vi "can_test.vi"() -> ()   [LabVIEW 2020]
uses:
  <vilib>/xnet/xnet.llb/XNET Frame CAN.ctl
  <vilib>/xnet/xnet.llb/XNET Frame Type CAN.ctl
  <vilib>/xnet/xnet.llb/XNET Create Session (Frame Output Stream).vi
  <vilib>/xnet/xnet.llb/XNET Write (Frame CAN).vi
  <resource>/objmgr/xnet.rc
panel:
  out "Array 2":T1[](array[typedef]) {"payload" format="%x"; "timestamp" format="%<%.7X\n%x>T"; "type" items=["CAN Data"=0, "CAN Remote"=1, "CAN Bus Error"=2, "CAN 2.0 Data"=8, "CAN FD Data"=16, "CAN FD+BRS Data"=24, "J1939 Data"=192, "Delay"=224, "Log Trigger"=225, "Start Trigger"=226]; "identifier" format="%x"}
  out "Array":T1[](array[typedef]) {"payload" format="%x"; "timestamp" format="%<%.7X\n%x>T"; "type" items=["CAN Data"=0, "CAN Remote"=1, "CAN Bus Error"=2, "CAN 2.0 Data"=8, "CAN FD Data"=16, "CAN FD+BRS Data"=24, "J1939 Data"=192, "Delay"=224, "Log Trigger"=225, "Start Trigger"=226]; "identifier" format="%x"}
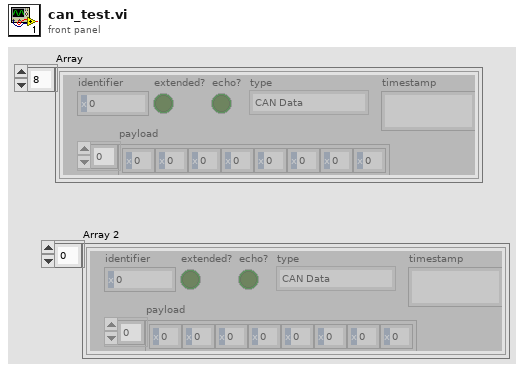
[diagram p1: front panel]
types:
  T1 = typedef "XNET Frame CAN.ctl" = cluster{"timestamp":timestamp, "payload":u8[], "identifier":u32, "type":T2, "extended?":bool, "echo?":bool}
  T2 = typedef "XNET Frame Type CAN.ctl" = u8
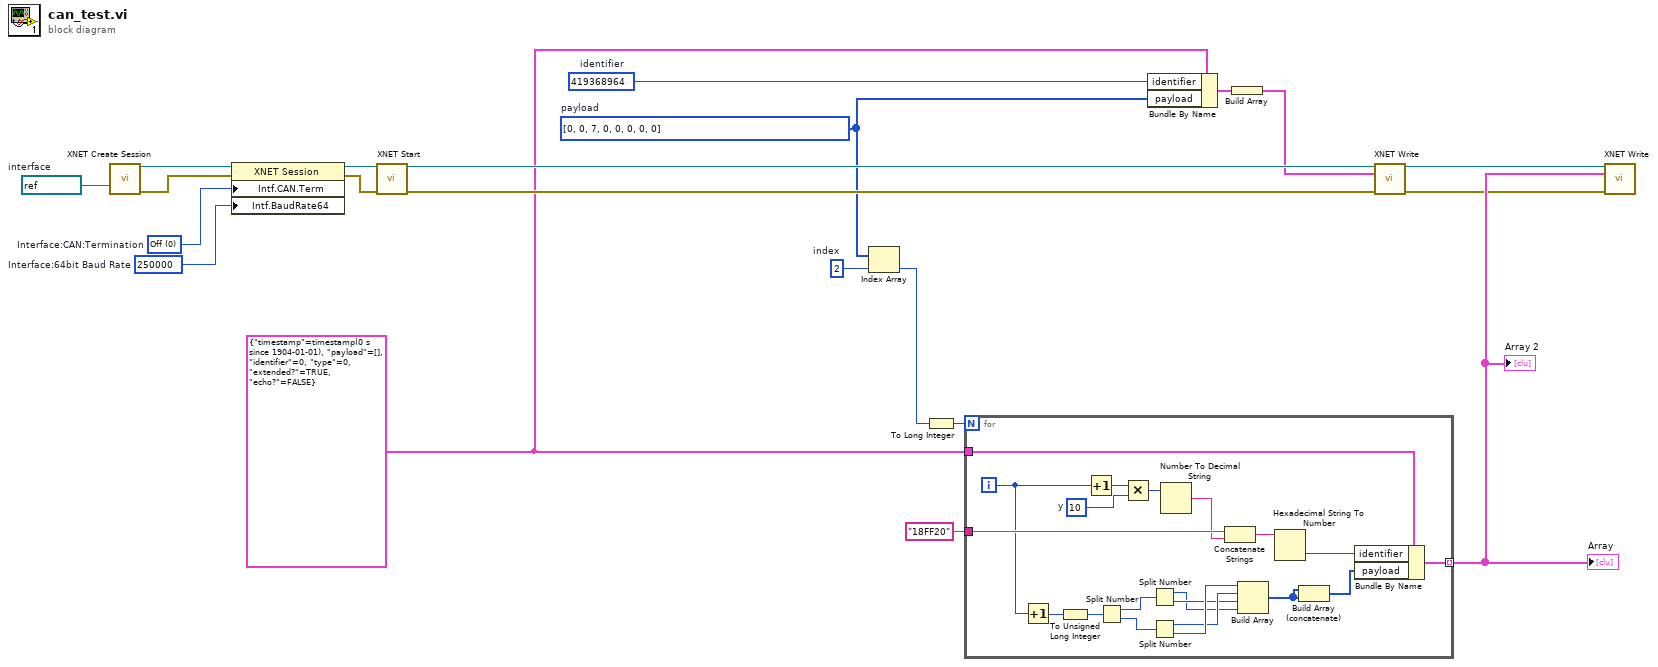
[diagram p0: block diagram]
diagram:
  w3 = 2  # index
  w4 = u8[] [0, 0, 7, 0, 0, 0, 0, 0]  # payload
  w7 = u32 419368964  # identifier
  w17 = u32 0 items=["Off", "On"]  # Interface:CAN:Termination
  w18 = u64 250000  # Interface:64bit Baud Rate
  w8 = T1 {"timestamp"=timestamp(0 s since 1904-01-01), "payload"=[], "identifier"=0, "type"=0, "extended?"=TRUE, "echo?"=FALSE} ("CAN frame")
  w21 = refnum<k21> "CAN1"  # interface
  n1 = call-poly <vilib>:"XNET Create Session.vi"("interface"=w21) -> ("session out"=w20:refnum<k21>, "error out"=w16:errorcluster)  [unwired: 13 in]
  n2 = property class="XNET Session"(reference=w20, error in=w16, "Intf.CAN.Term"=w17, "Intf.BaudRate64"=w18) -> (reference out=w19:refnum<k21>, error out=w15:errorcluster)
  n3 = call <vilib>:"XNET Start.vi"("session in"=w19, "error in (no error)"=w15) -> ("session out"=w10:refnum<k21>, "error out"=w12:errorcluster)  [unwired: 12 in]
  n4 = Index Array(array=w4, index=w3) -> (element=w2:u8)
  n5 = To Long Integer(number=w2) -> (32bit integer=w1:i32)
  n6 = for {
    N: w1 -> [_]
    tunnel: w8 -> [w41]
    tunnel: [w39] -> w14 mode=indexing
    tunnel: "18FF20" -> [w37]
    i -> [w32]
    w40 = 10  # y
    n7 = Increment(x=w32) -> (x+1=w22:i32)
    n8 = To Unsigned Long Integer(number=w22) -> (unsigned 32bit integer=w31:u32)
    n9 = Increment(x=w32) -> (x+1=w33:i32)
    n10 = Split Number(x=w31) -> (hi(x)=w30:u16, lo(x)=w29:u16)
    n11 = Multiply(x=w33, y=w40) -> (x*y=w38:i32)
    n12 = Split Number(x=w30) -> (hi(x)=w23:u8, lo(x)=w24:u8)
    n13 = Split Number(x=w29) -> (hi(x)=w25:u8, lo(x)=w26:u8)
    n14 = Number To Decimal String(number=w38) -> (decimal integer string=w36:string)  [unwired: 1 in]
    n15 = Concatenate Strings(w37, w36) -> (w35:string)
    n16 = Build Array(w26, w25, w24, w23) -> (w28:u8[])
    n17 = Hexadecimal String To Number(string=w35) -> (number=w34:u32)  [unwired: 2 in, 1 out]
    n18 = Build Array (concatenate)(w28, w28) -> (w27:u8[])
    n19 = Bundle By Name(cluster=w41, "identifier"=w34, "payload"=w27) -> (w39:T1)
  }
  "Array" <- w14
  "Array 2" <- w14
  n20 = Bundle By Name(cluster=w8, "identifier"=w7, "payload"=w4) -> (w6:T1)
  n21 = Build Array(w6) -> (w5:T1[])
  n22 = call-poly <vilib>:"XNET Write.vi"("session in"=w10, "data"=w5, "error in (no error)"=w12) -> ("session out"=w9:refnum<k21>, "error out"=w11:errorcluster)  [unwired: 11 in]
  n23 = call-poly <vilib>:"XNET Write.vi"("session in"=w9, "data"=w14, "error in (no error)"=w11) -> ()  [unwired: 11 in, 2 out]
